vi "Dashboard Main.vi"() -> ()   [LabVIEW 2015]
uses:
  <vilib>/Utility/miscctls.llb/LVRowAndColumnTypeDef.ctl
  <vilib>/event_ctls.llb/eventvkey.ctl
  <vilib>/Rock Robotics/WPI/Dashboard/WPI_DashboardLogging Global.vi
  <vilib>/Rock Robotics/Network Tables/NT Read Numeric Array.vi
  <vilib>/Utility/config.llb/Write Key (String).vi
  <vilib>/Utility/config.llb/Write Key (I32).vi
  <vilib>/Utility/config.llb/NI_LVConfig.lvlib
panel:
  in  "TCP":refnum<k5>
  in  "Rec Mode":enum32{"Stop", "Record", "Playback"}(radio)
  in  "Vision":u16(ring) items=["Camera Off", "USB Camera SW", "USB Camera HW", "IP Camera"]
  out "Camera IP":string
  out "Image Message":string="Timeout in Camera Communications"
  in  "Dashboard Tab":T1(tab)
  out "dist":dbl
  in  "Select Auto":string(combo)
  out "NT Connection":bool
  in  "Camera Settings":T2={"Frame Rate"=30, "Compression"=30, "Size"=1} {"Frame Rate" scale=1.0..30.0; "Size" items=["640x480", "320x240", "160x120"]}
  out "MotorChart R":cluster{"Numeric":dbl, "Numeric":dbl}(graph)
  out "MotorChart L":T3(graph)
  out "MotorSliders R":cluster{"MotorSlide1":dbl, "MotorSlide2":dbl} {"MotorSlide2" scale=-1.0..1.0 scale format="%#_2e"; "MotorSlide1" scale=-1.0..1.0 scale format="%#_2e"}
  out "MotorSliders L":T4 {"MotorSlide4 2" scale=0.0..14.0 scale format="%#_2e"; "MotorSlide2" scale=-1.0..1.0 scale format="%#_2e"; "MotorSlide1" scale=-1.0..1.0 scale format="%#_2e"}
  out "Gyro":dbl(knob) scale=0.0..360.0
  out "JS1 Z":dbl(slide) scale=-1.0..1.0 scale format="%#_2e"
  out "JS1 Graph":cluster{"X":dbl, "Y":dbl}[](graph)
  out "JS1 Buttons":T5
  out "JS2 Z":dbl(slide) scale=-1.0..1.0 scale format="%#_2e"
  out "JS2 Graph":cluster{"X":dbl, "Y":dbl}[](graph)
  out "JS2 Buttons":T5
  out "Mode":T6(ring)=enum."Auto Disabled"
  in  "DB Camera Config":bool
  out "fps":dbl format="%#.1g"
  out "Mbps":dbl format="%#.1g"
  out "Mbps LED":bool
  in  "DB/String 9":string
  in  "DB/String 8":string
  in  "DB/String 7":string
  in  "DB/String 6":string
  in  "DB/String 5":string
  in  "DB/String 4":string
  in  "DB/String 3":string
  in  "DB/String 2":string
  in  "DB/String 1":string
  in  "DB/String 0":string
  in  "DB/Slider 0":dbl(slide) scale=0.0..5.0
  in  "DB/Slider 1":dbl(slide) scale=0.0..5.0
  in  "DB/Slider 2":dbl(slide) scale=0.0..5.0
  in  "DB/Slider 3":dbl(slide) scale=0.0..5.0
  out "DB/LED 3":bool
  out "DB/LED 2":bool
  out "DB/LED 1":bool
  out "DB/LED 0":bool
  in  "DB/Button 3":bool
  in  "DB/Button 2":bool
  in  "DB/Button 1":bool
  in  "DB/Button 0":bool caption="New Name"
  in  "Test Slider":dbl(slide) scale=0.0..100.0 scale format="%#_3g"
  in  "On/Off":bool caption="Solenoid"
  in  "Test Name":u16(ring) items=["Select the test to run..."]
  in  "Test Tree":string(tree)
  in  "Motor":cluster{"Value":dbl, "Enable":bool} {"Value" scale=-1.0..1.0 scale format="%#_3g"}
  out "Progress":T7 {"Test Progress" scale=0.0..100.0}
  in  "Rev/Fwd":cluster{"Forward":bool, "Reverse":bool}
  in  "Test Ring":u16(ring) items=["Monochrome", "Color"]
  out "Cmd Status":string
  in  "Execute Command":bool
  in  "Command Params":string[][](table)
  in  "Command Selection":i32(listbox)
  in  "CheckList":i32(listbox)
  out "Tree":string(tree)
  out "Camera Image":T8(plugin-control)
  out "Background":bool
  # "Left"
  # "Front"
  # "Right"
  # "Battery"
  # "This tab is a great place for autonomous settings and robot-specific values.\nPlace controls and indicators inside this tab and match name to\nDashboard Variables on robot. You can also delete this comment."
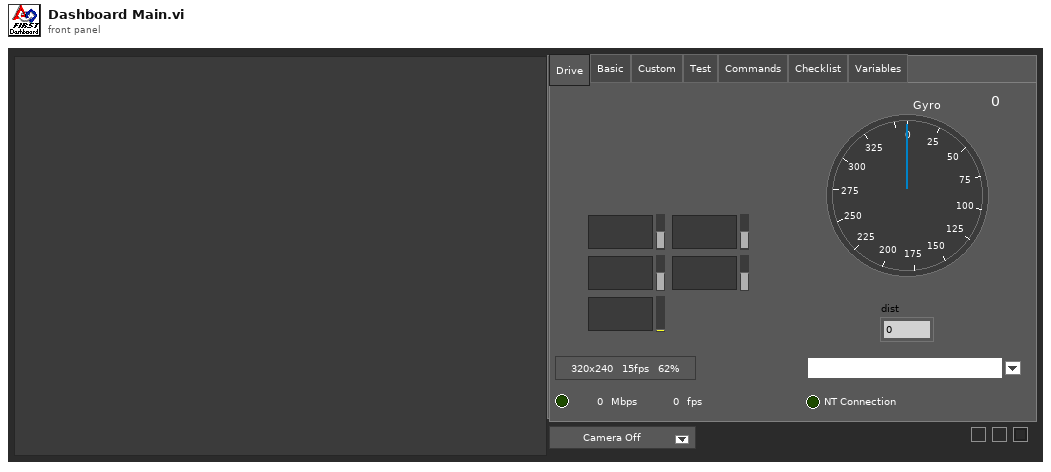
[diagram p1: front panel]
types:
  T1 = enum32{"Drive", "Basic", "Custom", "Test", "Commands", "Checklist", "Variables"}
  T2 = cluster{"Frame Rate":i32, "Compression":i32, "Size":u16}
  T3 = cluster{"Numeric":dbl, "Numeric":dbl, "Battery V":dbl}
  T4 = cluster{"MotorSlide1":dbl, "MotorSlide2":dbl, "MotorSlide4 2":dbl}
  T5 = cluster{bool, bool, bool, bool, bool, bool, bool, bool, bool, bool, bool, bool}
  T6 = enum8{"Tele-Op Disabled", "Tele-Op Enabled", "Auto Disabled", "Auto Enabled", "Test Disabled", "Test Enabled", "Disconnected", "No Code", "E-Stop"}
  T7 = cluster{"Test Progress":u8, "Test Progress Text":string}
  T8 = typedef "IMAQ Image.ctl" = refnum<image>
  T9 = cluster{"IDs":cluster{"RPC field ID":u16, "Unique ID":u16}, "String":string}
  T10 = enum32{"Drive", "Basic", "Custom", "Test", "Checklist", "Variables"}
  T11 = typedef "Image Type" = u32
  T12 = cluster{"Camera Image":refnum<vi>, "Dashboard Tab":refnum<vi>, "Background":refnum<vi>, "Vision":refnum<vi>, "Rec Mode":refnum<vi>, "Test Slider":refnum<vi>, "On/Off ":refnum<vi>, "Test Ring":refnum<vi>, "Rev/Fwd":refnum<vi>, "Test Name":refnum<vi>, "Motor":refnum<vi>, "Progress":refnum<vi>, "CheckList":refnum<vi>, "Tree":refnum<vi>, "Test Tree":refnum<vi>, "Command Params":refnum<vi>, "Command Selection":refnum<vi>, "Execute Command":refnum<vi>, "Cmd Status":refnum<vi>}
  T13 = cluster{"Error Strings":string, "Disable Counts":cluster{u16, u16}, "Rail Faults":cluster{u16, u16, u16}, "Robot IP":string, "DB Mode":u8, "Event Info":cluster{"Name":string, "Type":u8, "Number":u16, "Replay":u8}, "Camera Addr":string}
  T14 = cluster{"Storage":cluster{"Disk Free":u64, "RAM Block":u32, "RAM free":u32}, "CPU Utilization":cluster{"CPU % ISR":sgl, "CPU % Time Crit":sgl, "CPU % Timed Str":sgl, "CPU % High":sgl, "CPU % Above":sgl, "CPU % Normal":sgl, "CPU % Low":sgl}, "CAN":cluster{"% Bus Utilization":sgl, "Bus Off Cnt":u32, "TX_FIFO Full Cnt":u32, "Receive Error Cnt":u8, "Transmit Error Cnt":u8}, "HID":cluster{"HID Outputs":u32, "Rumble Low":u16, "Rumble High":u16}[]}
  T15 = cluster{"Status bits":cluster{"Test Mode":bool, "Autonomous":bool, "Enabled":bool, "Code Start":bool, "Brownout":bool, "Reserved 2":bool, "Reserved 3":bool, "E-Stop":bool}, "Code Trace":cluster{"Disabled":bool, "TeleOp":bool, "Auto":bool, "Test":bool}, "Controller Type":enum16{"unknown", "cRIO", "roboRio"}, "Code?":enum16{"unknown", "noCode", "code"}, "Battery V":dbl}
  T16 = cluster{"Control Bits":cluster{"TestMode":bool, "Autonomous":bool, "Enabled":bool, "FMS Present":bool, bool, bool, bool, "E-Stop":bool}, "Team Station ":u8, "Countdown":sgl, "Joystick Values":cluster{"Axes":dbl[], "Buttons":bool[], "POVs":i16[]}[]}
  T17 = cluster{"Axes":dbl[], "Buttons":bool[], "POVs":i16[]}[]
  T18 = cluster{"Axes":dbl[], "Buttons":bool[], "POVs":i16[]}
  T19 = cluster{"Buttons[0]":bool, "Buttons[1]":bool, "Buttons[2]":bool, "Buttons[3]":bool, "Buttons[4]":bool, "Buttons[5]":bool, "Buttons[6]":bool, "Buttons[7]":bool, "Buttons[8]":bool, "Buttons[9]":bool, "Buttons[10]":bool, "Buttons[11]":bool}
  T20 = typedef "NI_LVConfig.lvlib/Config Data RefNum.ctl" = refnum<k1>
  T21 = cluster{"Operation":enum16{"Update", "Clear"}, "Color Box":u32}[]
  T22 = typedef "eventvkey.ctl" = enum16{"ASCII", "Enter", "Return", "Shift", "Ctrl", "Alt", "Cmd", "Opt", "Caps", "NumLock", "Clear", "Break", "Up", "Down", "Left", "Right", "Insert", "Delete", "Home", "End", "PageUp", "PageDown", "Escape", "Help", "Pause", "ScrollLock", "F1", "F2", "F3", "F4", "F5", "F6", "F7", "F8", "F9", "F10", "F11", "F12", "F13", "F14", "F15", "F16", "F17", "F18", "F19", "F20", "F21", "F22", "F23", "F24", "Play", "VolumeUp", "VolumeDown", "Mute", "Two Byte Char"}
  T23 = cluster{"Image Size":bool, "Image Type":bool, "Pixel Value":bool, "ROI Information":bool, "Zoom Factor":bool}
  T24 = enum8{"Enabled", "Disabled", "Disabled and Grayed Out"}
  T25 = cluster{"Operation":enum16{"Update", "Clear"}, "Color Box":u32}
  T26 = typedef "LVRowAndColumnTypeDef.ctl" = cluster{"Row":i32, "Column":i32}
  T27 = cluster{"Shift":bool, "Ctrl":bool, "Alt":bool, "Cmd":bool, "Opt":bool}
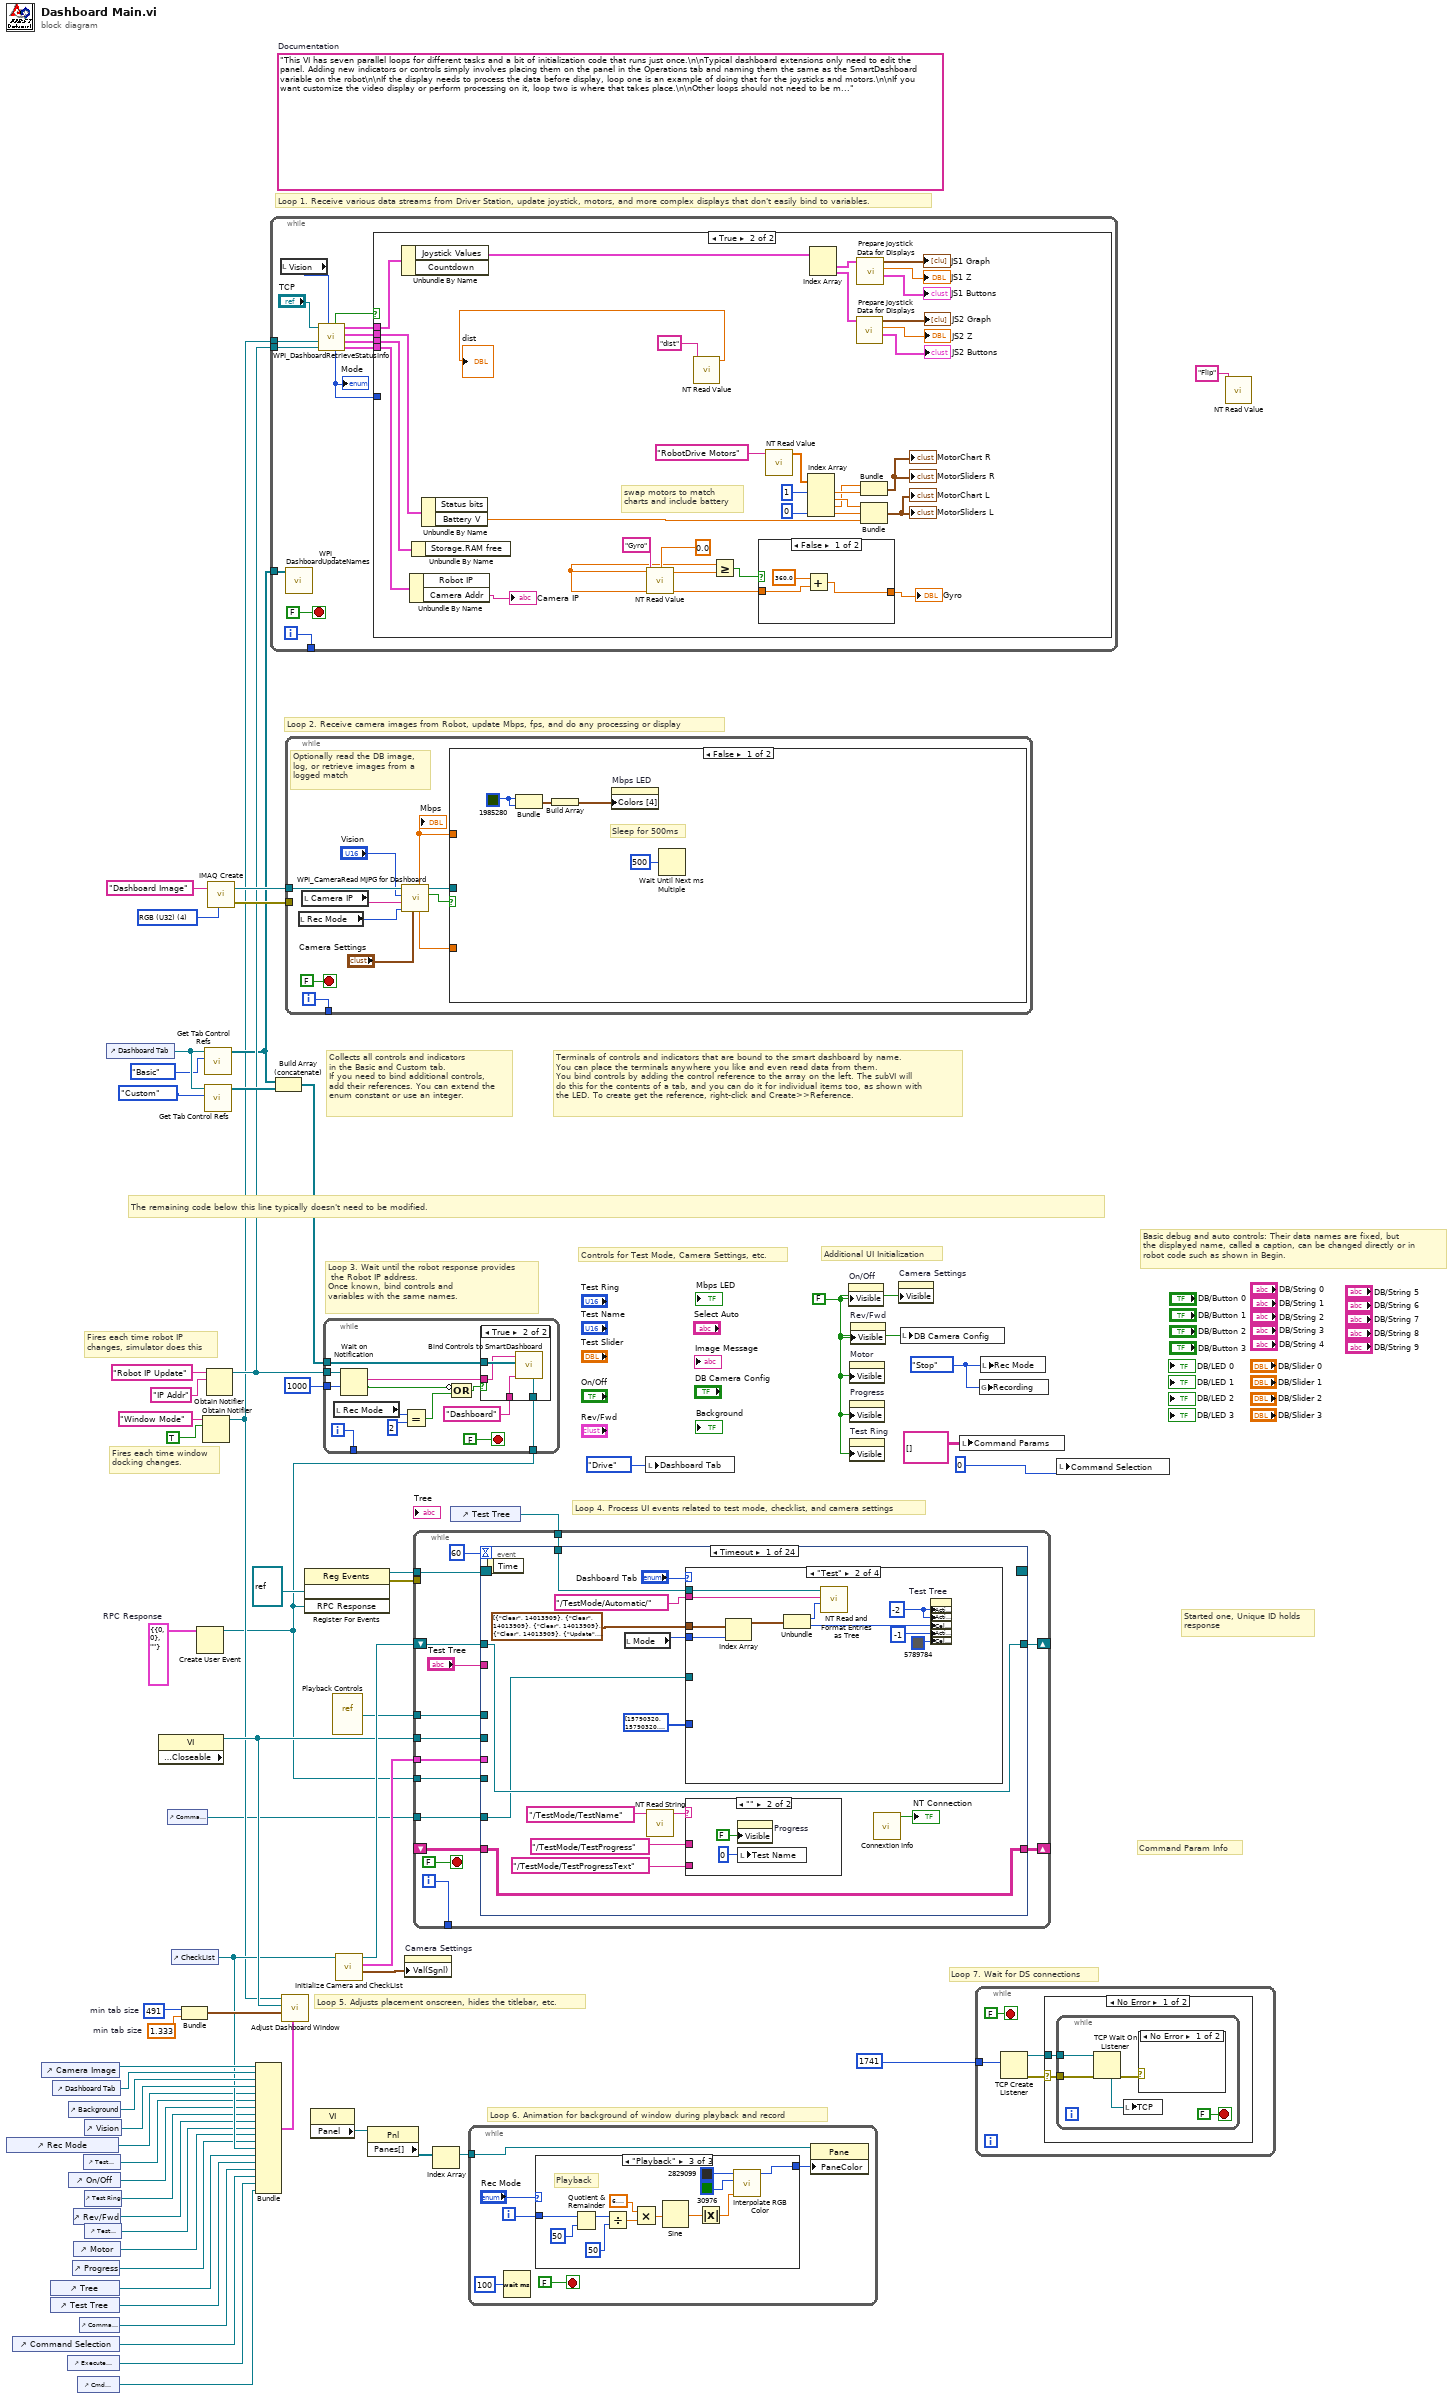
[diagram p0: block diagram]
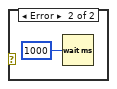
[diagram p2: hidden frame]
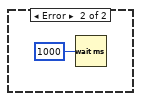
[diagram p3: hidden frame]
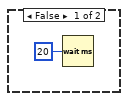
[diagram p4: hidden frame]
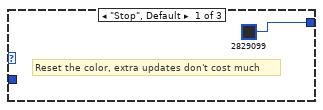
[diagram p6: hidden frame]
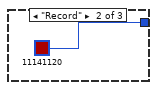
[diagram p7: hidden frame]
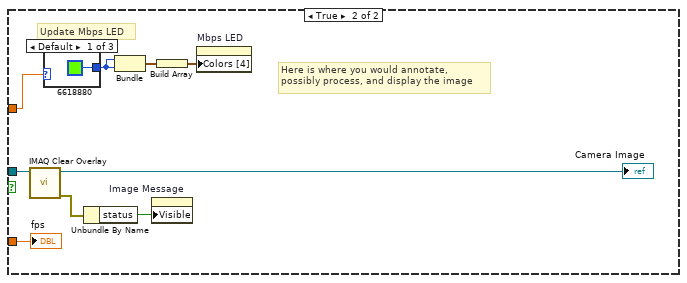
[diagram p9: hidden frame]
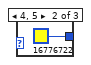
[diagram p10: hidden frame]
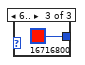
[diagram p11: hidden frame]
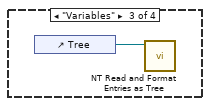
[diagram p13: hidden frame]
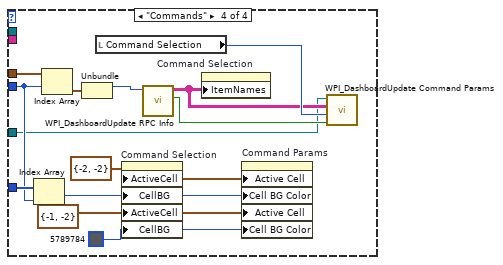
[diagram p14: hidden frame]
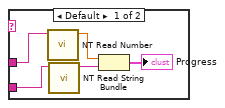
[diagram p15: hidden frame]
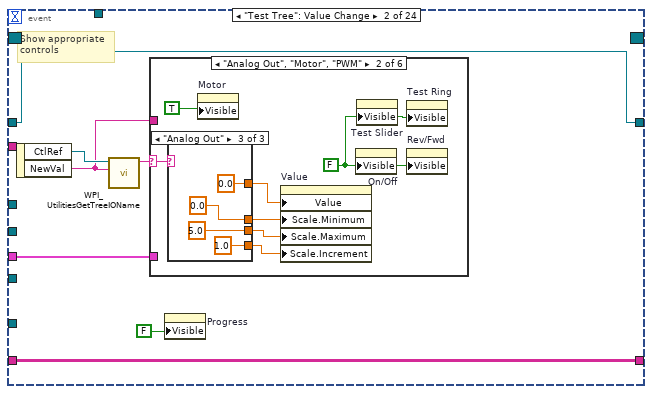
[diagram p16: hidden frame]
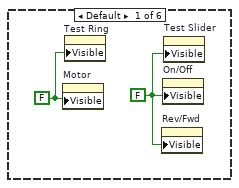
[diagram p17: hidden frame]
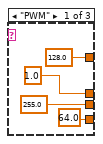
[diagram p18: hidden frame]
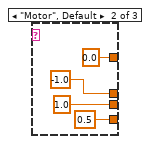
[diagram p19: hidden frame]
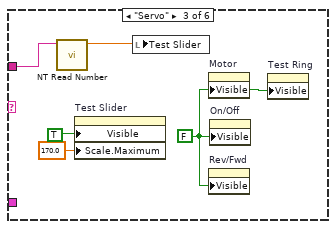
[diagram p20: hidden frame]
diagram:
  w8 = T9 {"IDs"={"RPC field ID"=0, "Unique ID"=0}, "String"=""}  # RPC Response
  w34 = 491  # min tab size
  w33 = 1.333  # min tab size
  w42 = enum32{"Stop", "Record", "Playback"}."Stop" ("Rec Mode")
  w16 = FALSE ("Visible")
  (unwired) "This VI has seven parallel loops for different tasks and a bit of initialization code that runs just once.\n\nTypical dashboard extensions only need to edit the panel. Adding new indicators or controls simply involves placing them on the panel in the Operations tab and naming them the same as the SmartDashboard variable on the robot\n\nIf the display needs to process the data before display, loop one is an example of doing that for the joysticks and motors.\n\nIf you want customize the video display or perform processing on it, loop two is where that takes place.\n\nOther loops should not need to be modified. They are pretty standard, and document the task they perform."  # Documentation
  w62 = T11 4 items=["Grayscale (U8)", "Grayscale (I16)", "Grayscale (SGL)", "Complex (CSG)", "RGB (U32)", "HSL (U32)", "RGB (U64)"] ("Image Type")
  # "Command Param Info"
  # "Started one, Unique ID holds\nresponse"
  # "Loop 7. Wait for DS connections"
  # "Basic debug and auto controls: Their data names are fixed, but\nthe displayed name, called a caption, can be changed directly or in\nrobot code such as shown in Begin."
  # "Controls for Test Mode, Camera Settings, etc."
  # "Additional UI Initialization"
  # "Loop 6. Animation for background of window during playback and record"
  # "Fires each time robot IP\nchanges, simulator does this"
  # "Fires each time window\ndocking changes."
  # "Collects all controls and indicators\nin the Basic and Custom tab.\nIf you need to bind additional controls,\nadd their references. You can extend the\nenum constant or use an integer."
  # "The remaining code below this line typically doesn't need to be modified."
  # "Loop 4. Process UI events related to test mode, checklist, and camera settings"
  # "Terminals of controls and indicators that are bound to the smart dashboard by name.\nYou can place the terminals anywhere you like and even read data from them.\nYou bind controls by adding the control reference to the array on the left. The subVI will\ndo this for the contents of a tab, and you can do it for individual items too, as shown with\nthe LED. To create get the reference, right-click and Create>>Reference."
  # "Loop 3. Wait until the robot response provides\n the Robot IP address.\nOnce known, bind controls and\nvariables with the same names."
  # "Loop 5. Adjusts placement onscreen, hides the titlebar, etc."
  # "Loop 1. Receive various data streams from Driver Station, update joystick, motors, and more complex displays that don't easily bind to variables."
  # "Loop 2. Receive camera images from Robot, update Mbps, fps, and do any processing or display"
  n1 = control-ref of="Rec Mode"() -> (w22:refnum<vi>)
  n2 = control-ref of="Command Selection"() -> (w7:refnum<vi>)
  n3 = control-ref of="Camera Image"() -> (w37:refnum<vi>)
  n4 = control-ref of="Tree"() -> (w26:refnum<vi>)
  n5 = control-ref of="Test Tree"() -> (w25:refnum<vi>)
  n6 = control-ref of="Dashboard Tab"() -> (w36:refnum<vi>)
  n7 = control-ref of="Execute Command"() -> (w9:refnum<vi>)
  n8 = control-ref of="Background"() -> (w31:refnum<vi>)
  n9 = control-ref of="On/Off"() -> (w20:refnum<vi>)
  n10 = control-ref of="Progress"() -> (w17:refnum<vi>)
  n11 = control-ref of="Rev/Fwd"() -> (w18:refnum<vi>)
  n12 = control-ref of="Motor"() -> (w23:refnum<vi>)
  n13 = control-ref of="Cmd Status"() -> (w3:refnum<vi>)
  n14 = control-ref of="Command Params"() -> (w10:refnum<vi>)
  n15 = control-ref of="Test Slider"() -> (w21:refnum<vi>)
  n16 = control-ref of="Vision"() -> (w35:refnum<vi>)
  n17 = control-ref of="Test Ring"() -> (w19:refnum<vi>)
  n18 = control-ref of="Test Name"() -> (w24:refnum<vi>)
  n19 = control-ref of="Dashboard Tab"() -> (w40:refnum<vi>)
  n20 = property class="VI" props=["Front Panel.Closeable"]() -> (reference out=w41:refnum<vi>)  [unwired: 2 in, 2 out]
  n21 = control-ref of="Command Params"() -> (w2:refnum<vi>)
  n22 = control-ref of="CheckList"() -> (w27:refnum<vi>)
  n23 = Bundle("min tab size"=w34, "min tab size"=w33) -> (w32:cluster{"min tab size":i32, "min tab size":dbl})  [unwired: 1 in]
  n24 = Create User Event(user event datatype=w8) -> (user event=w4:refnum<user-event>)  [unwired: 1 in, 1 out]
  n25 = Obtain Notifier(name (unnamed)="Window Mode", notification data type=TRUE) -> (notifier out=w13:refnum<notifier>)  [unwired: 2 in, 2 out]
  n26 = call <vilib>:"Get Tab Control Refs.vi"("Page Index"=T10."Basic" ("Dashboard Tab"), "TabControl in"=w40) -> ("ControlsOnPage"=w14:refnum<vi>[])  [unwired: 9 in]
  n27 = call <vilib>:"Get Tab Control Refs.vi"("Page Index"=T10."Custom" ("Dashboard Tab"), "TabControl in"=w40) -> ("ControlsOnPage"=w39:refnum<vi>[])  [unwired: 9 in]
  n28 = Obtain Notifier(name (unnamed)="Robot IP Update", notification data type="IP Addr" ("name (unnamed)")) -> (notifier out=w15:refnum<notifier>)  [unwired: 2 in, 2 out]
  n29 = call "IMAQ Create"("Image Name"="Dashboard Image", "Image Type"=w62) -> ("New Image"=w60:T8, "error out"=w59:errorcluster)  [unwired: 2 in, 1 out]
  n30 = Bundle("Camera Image"=w37, "Dashboard Tab"=w36, "Background"=w31, "Vision"=w35, "Rec Mode"=w22, "Test Slider"=w21, "On/Off"=w20, "Test Ring"=w19, "Rev/Fwd"=w18, "Test Name"=w24, "Motor"=w23, "Progress"=w17, "CheckList"=w27, "Tree"=w26, "Test Tree"=w25, "Command Params"=w10, "Command Selection"=w7, "Execute Command"=w9, "Cmd Status"=w3) -> (w28:T12)  [unwired: 1 in]
  n31 = while {
    tunnel: [w74] -> _
    tunnel: w15 -> [w68]
    tunnel: w14 -> [w67]
    tunnel: w13 -> [w63]
    i -> [w74]
    stop <- FALSE stop-if-true
    n32 = local read "Vision"() -> (w65:u16)
    n33 = call <vilib>:"WPI_DashboardUpdateNames.vi"("Controls on Tab"=w67) -> ()  [unwired: 11 in]
    n34 = call <vilib>:"WPI_DashboardRetrieveStatusInfo.vi"("Vision"=w65, "Binding Refnum"=w68, "Window Mode Notifier"=w63, "TCP Cnx"="TCP") -> ("Power and Errors"=w69:T13, "Robot Metrics"=w72:T14, "Status Info"=w73:T15, "Control Info"=w70:T16, "Robot Mode"=w66:T6, "Process?"=w71:bool)  [unwired: 2 in]
    "Mode" <- w66
    n35 = case shown="True" w71 {
      tunnel: w73 -> [_ w108]
      tunnel: w72 -> [_ w107]
      tunnel: w70 -> [_ w106]
      tunnel: w69 -> [_ w105]
      tunnel: w66 -> [_ _]
      frame False {
        n36 = Wait (ms)(milliseconds to wait=u32 20) -> ()  [unwired: 1 out]
      }
      frame True {
        # "swap motors to match\ncharts and include battery"
        n37 = Unbundle By Name(w106) -> ("Joystick Values"=w95:T17)  [unwired: 1 out]
        n38 = Unbundle By Name(w105) -> ("Camera Addr"=→"Camera IP":string)  [unwired: 1 out]
        n39 = Unbundle By Name(w107) -> ()  [unwired: 1 out]
        n40 = Unbundle By Name(w108) -> ("Battery V"=w96:dbl)  [unwired: 1 out]
        n41 = call-poly <vilib>:"NT Read Value.vi"("Name"="Gyro") -> ("Numeric"=w80:dbl)  [unwired: 9 in, 1 out]
        n42 = call-poly <vilib>:"NT Read Value.vi"("Name"="dist") -> ("Numeric"=→"dist":dbl)  [unwired: 9 in, 1 out]
        n43 = Greater Or Equal?(x=w80, y=0.0) -> (x >= y?=w82:bool)
        n44 = case shown="False" w82 {
          tunnel: [w109 w112] -> w79
          tunnel: w80 -> [w110 w112]
          frame False {
            n45 = Add(x=360.0, y=w110) -> (x+y=w109:dbl)
          }
          frame True {
          }
        }
        "Gyro" <- w79
        n46 = call-poly <vilib>:"NT Read Value.vi"("Name"="RobotDrive Motors") -> ("Numeric Array"=w84:dbl[])  [unwired: 9 in, 1 out]
        n47 = Index Array(array=w84, index #1=1, index #4=0) -> (element #1=w100:dbl, element #2=w101:dbl, element #3=w99:dbl, element #4=w104:dbl)  [unwired: 2 in]
        n48 = Index Array(array=w95) -> (element #1=w94:T18, element #2=w89:T18)  [unwired: 2 in]
        n49 = call "Prepare Joystick Data for Displays.vi"("Joystick Values"=w89) -> ("Buttons"=→"JS2 Buttons":T19, "Z Axis"=→"JS2 Z":dbl, "Cartesian Data"=→"JS2 Graph":cluster{"X axis":dbl, "X axis":dbl}[])  [unwired: 8 in]
        n50 = call "Prepare Joystick Data for Displays.vi"("Joystick Values"=w94) -> ("Buttons"=→"JS1 Buttons":T19, "Z Axis"=→"JS1 Z":dbl, "Cartesian Data"=→"JS1 Graph":cluster{"X axis":dbl, "X axis":dbl}[])  [unwired: 8 in]
        n51 = Bundle("Numeric"=w99, "Numeric"=w100) -> (→"MotorChart R" →"MotorSliders R":cluster{"Numeric":dbl, "Numeric":dbl})  [unwired: 1 in]
        n52 = Bundle("Numeric"=w101, "Numeric"=w104, "Battery V"=w96) -> (→"MotorChart L" →"MotorSliders L":T3)  [unwired: 1 in]
      }
    }
  }
  n53 = Build Array (concatenate)(w14, w39) -> (w38:refnum<vi>[])
  n54 = call "Adjust Dashboard Window.vi"("Sizing Refnums"=w28, "Size Constraints"=w32, "VI"=w41, "WIn Mode"=w13) -> ()  [unwired: 8 in]
  n55 = while {
    tunnel: w60 -> [w121]
    tunnel: w59 -> [_]
    tunnel: [w122] -> _
    i -> [w122]
    stop <- FALSE stop-if-true
    # "Optionally read the DB image,\nlog, or retrieve images from a\nlogged match"
    n56 = local read "Rec Mode"() -> (w116:enum32{"Stop", "Record", "Playback"})
    n57 = local read "Camera IP"() -> (w114:string)
    n58 = call <vilib>:"WPI_CameraRead MJPG for Dashboard.vi"("Camera Settings"="Camera Settings", "Rec Mode"=w116, "Camera IP"=w114, "Camera Mode"="Vision", "Refnum in"=w121) -> ("Active"=w119:bool, "Refnum out"=w120:T8, "FPS"=w118:dbl, "Bandwidth (Mbps)"=w113:dbl)  [unwired: 3 in]
    "Mbps" <- w113
    n59 = case shown="False" w119 {
      tunnel: w120 -> [_ w131]
      tunnel: w113 -> [_ w130]
      tunnel: w118 -> [_ w128]
      frame False {
        w124 = u32 1985280 ("Color Box")
        # "Sleep for 500ms"
        n60 = Bundle("Color Box"=w124, "Color Box"=w124) -> (w126:cluster{"Color Box":u32, "Color Box":u32})  [unwired: 1 out]
        n61 = Build Array(w126) -> (w125:cluster{"Color Box":u32, "Color Box":u32}[])
        n62 = property on="Mbps LED" class="Bool (strict)"("Colors [4]"=w125) -> ()  [unwired: 2 in, 2 out]
        n63 = Wait Until Next ms Multiple(millisecond multiple=u32 500) -> ()  [unwired: 1 out]
      }
      frame True {
        # "Here is where you would annotate,\npossibly process, and display the image"
        # "Update Mbps LED"
        n64 = call "IMAQ Clear Overlay"("Image"=w131) -> ("error out"=w135:errorcluster, "Image Out"=→"Camera Image":T8)  [unwired: 2 in, 7 out]
        n65 = case shown="Default" w130 {
          tunnel: [u32 6618880 ("Color Box") u32 16776722 ("Color Box") u32 16716800 ("Color Box")] -> w132
          frame Default {
          }
          frame 4, 5 {
          }
          frame 6.. {
          }
        }
        n66 = Unbundle By Name(w135) -> ("status"=w136:bool)
        n67 = Bundle("Color Box"=w132, "Color Box"=w132) -> (w134:cluster{"Color Box":u32, "Color Box":u32})  [unwired: 1 out]
        n68 = property on="Image Message" class="Str"("Visible"=w136) -> ()  [unwired: 2 in, 2 out]
        n69 = Build Array(w134) -> (w133:cluster{"Color Box":u32, "Color Box":u32}[])
        n70 = property on="Mbps LED" class="Bool (strict)"("Colors [4]"=w133) -> ()  [unwired: 2 in, 2 out]
        "fps" <- w128
      }
    }
  }
  n71 = register-events(refnum<vi> refnum, w4) -> (reference out=w46:refnum<event-registration>, error out=w45:errorcluster)  [unwired: 2 in]
  n72 = property class="VI"() -> ("Panel"=w49:refnum<vi>)  [unwired: 2 in, 2 out]
  n73 = while {
    tunnel: w38 -> [w152]
    tunnel: w15 -> [w150]
    tunnel: [w148] -> _
    tunnel: u32 1000 ("milliseconds to wait") -> [w147]
    tunnel: w4 -> [w140]
    i -> [w148]
    stop <- FALSE stop-if-true
    n74 = local read "Rec Mode"() -> (w143:enum32{"Stop", "Record", "Playback"})
    n75 = Wait on Notification(notifier=w150, timeout in ms (-1)=w147) -> (notification=w149:string, timed out?=w145:bool)  [unwired: 2 in, 2 out]
    n76 = Equal?(x=w143, y=u16 2 ("Rec Mode")) -> (x = y?=w144:bool)
    n77 = Compound Arithmetic op=OR(invert w145, w144) -> (w146:bool)
    n78 = case shown="True" w146 {
      tunnel: w152 -> [_ w156]
      tunnel: w149 -> [_ w155]
      tunnel: "Dashboard" -> [_ w154]
      tunnel: w140 -> [_ w153]
      frame False {
      }
      frame True {
        n79 = call <vilib>:"Bind Controls to SmartDashboard.vi"("RPC ref"=w153, "Client Name"=w154, "Bound Control Refs"=w156, "Server IP Address"=w155) -> ()  [unwired: 8 in]
      }
    }
  }
  n80 = vi-ref "Playback Controls.vi"() -> (w47:refnum<vi>)
  n81 = call "Initialize Camera and CheckList.vi"("ListBox in"=w27) -> ("Cluster"=w53:cluster{"value":i32, "value":i32, "index":i32}, "Array"=w54:cluster{string[]}[], "File Refnum"=w52:T20)  [unwired: 8 in]
  n82 = property class="Pnl"(reference=w49) -> ("Panes[]"=w50:refnum<vi>[])  [unwired: 1 in, 2 out]
  n83 = property on="Camera Settings" class="Clust (strict)"("Val(Sgnl)"=w53) -> ()  [unwired: 2 in, 2 out]
  n84 = Index Array(array=w50) -> (element=w48:refnum<vi>)  [unwired: 1 in]
  n85 = control-ref of="Test Tree"() -> (w51:refnum<vi>)
  n86 = while {
    tunnel: w54 -> [w168]
    shift-right: [w167] -> _
    shift-left: w52 -> [w166]
    tunnel: [w165] -> _
    tunnel: w51 -> [w164]
    tunnel: w47 -> [w163]
    tunnel: w46 -> [w162]
    tunnel: w45 -> [_]
    tunnel: w41 -> [w161]
    tunnel: w4 -> [w160]
    tunnel: w2 -> [w159]
    shift-right: [w158] -> _
    shift-left: _ -> [w157]
    i -> [w165]
    stop <- FALSE stop-if-true
    n87 = event shown="[0] Timeout" {
      selector: w162 -> [_ _ _ _ _ _ _ _ _ _ _ _ _ _ _ _ _ _ _ _ _ _ _ _]
      dyn-events: [_ _ _ _ _ _ _ _ _ _ _ _ _ _ _ _ _ _ w477 _ _ _ _ _] -> _
      timeout: u32 60 ("milliseconds to wait") -> [_ _ _ _ _ _ _ _ _ _ _ _ _ _ _ _ _ _ _ _ _ _ _ _]
      tunnel: w164 -> [w181 _ _ _ _ _ _ _ _ _ _ _ _ _ _ _ _ _ _ _ _ _ _ _]
      tunnel: "Test Tree" -> [_ _ _ _ _ _ _ _ _ _ _ _ _ w440 w449 w452 w457 w466 _ _ _ _ _ _]
      tunnel: w168 -> [_ w219 _ _ _ _ _ _ _ _ _ w402 w433 _ _ _ _ _ _ _ _ _ _ _]
      tunnel: [w178 w218 w322 w328 w338 w342 w348 w360 w368 w374 w387 w401 w426 w439 w447 w451 w456 w465 w479 w495 w497 w505 w516 w521] -> w167
      tunnel: w166 -> [w178 w218 w322 w328 w338 w342 w348 w360 w368 w374 w387 w400 w426 w439 w447 w451 w456 w465 w479 w495 w497 w505 w516 w521]
      tunnel: w163 -> [_ _ _ _ _ _ _ _ _ _ _ _ _ _ _ _ _ _ w480 _ w500 _ _ _]
      tunnel: w161 -> [_ _ _ _ _ _ _ _ _ _ _ _ _ _ _ _ _ _ w475 _ _ _ _ _]
      tunnel: w160 -> [_ _ _ _ _ _ _ _ _ _ _ _ _ _ _ _ _ _ w471 _ _ _ _ _]
      tunnel: w159 -> [w173 _ _ _ _ _ w346 _ _ _ _ _ _ _ _ _ _ _ _ _ _ _ _ _]
      tunnel: [w172 w217 w321 w327 w337 w343 w344 w354 w365 w373 w386 w399 w425 w438 w446 w450 w455 w464 w470 w493 w496 w501 w509 w522] -> w158
      tunnel: w157 -> [w172 w217 w321 w327 w337 w343 w344 _ _ w373 w386 w399 w425 w438 w446 w450 w455 w464 w470 w493 w496 w501 w509 w522]
      event Timeout {
        n88 = event-data() -> ()  [unwired: 1 in, 1 out]
        n89 = local read "Mode"() -> (w175:T6)
        n90 = call <vilib>:"NT Read String.vi"("Name"="/TestMode/TestName") -> ("String"=w184:string)  [unwired: 9 in, 1 out]
        n91 = case shown="\"Test\"" "Dashboard Tab" {
          tunnel: w181 -> [_ w195 _ _]
          tunnel: "/TestMode/Automatic/" ("Name Pattern") -> [_ w194 _ _]
          tunnel: T21 [{"Operation"=enum."Clear", "Color Box"=14013909}, {"Operation"=enum."Clear", "Color Box"=14013909}, {"Operation"=enum."Clear", "Color Box"=14013909}, {"Operation"=enum."Clear", "Color Box"=14013909}, {"Operation"=enum."Update", "Color Box"=14013909}, {"Operation"=enum."Update", "Color Box"=16777215}, {"Operation"=enum."Clear", "Color Box"=14013909}, {"Operation"=enum."Clear", "Color Box"=14013909}, {"Operation"=enum."Clear", "Color Box"=14013909}] -> [_ w187 _ w204]
          tunnel: w175 -> [_ w186 _ w203]
          tunnel: u32[] [15790320, 15790320, 15790320, 15790320, 16777215, 16777215, 15790320, 15790320, 15790320] -> [_ _ _ w209]
          tunnel: w173 -> [_ _ _ w197]
          frame "Custom", Default {
          }
          frame "Test" {
            w193 = -2 ("Active Item:Row Number")
            n92 = Index Array(array=w187, index=w186) -> (element=w188:T25)
            n93 = Unbundle(w188) -> ("Operation"=w189:enum16{"Update", "Clear"}, "Color Box"=w190:u32)
            n94 = call <vilib>:"NT Read and Format Entries as Tree.vi"("Operation"=w189, "Name Pattern"=w194, "Tree Refnum"=w195) -> ()  [unwired: 7 in, 2 out]
            n95 = property on="Test Tree" class="Tree (strict)"("Active Item Row Number"=w193, "ActiveColNum"=w193, "CellBG"=w190, "Active Item Row Number"=-1 ("Active Item:Row Number"), "CellBG"=u32 5789784 ("Color Box")) -> ()  [unwired: 2 in, 2 out]
          }
          frame "Variables" {
            n96 = control-ref of="Tree"() -> (w196:refnum<vi>)
            n97 = call <vilib>:"NT Read and Format Entries as Tree.vi"("Tree Refnum"=w196) -> ()  [unwired: 9 in, 2 out]
          }
          frame "Commands" {
            w205 = u32 5789784 ("Color Box")
            w206 = T26 {"Row"=-1, "Column"=-2} ("Active Cell:Active Cell")
            w208 = T26 {"Row"=-2, "Column"=-2} ("Active Cell:Active Cell")
            n98 = Index Array(array=w209, index=w203) -> (element=w207:u32)
            n99 = Index Array(array=w204, index=w203) -> (element=w202:T25)
            n100 = Unbundle(w202) -> ("Operation"=w201:enum16{"Update", "Clear"})  [unwired: 1 out]
            n101 = local read "Command Selection"() -> (w200:i32)
            n102 = property on="Command Selection" class="MCListbox (strict)"("ActiveCell"=w208, "CellBG"=w207, "ActiveCell"=w206, "CellBG"=w205) -> ()  [unwired: 2 in, 2 out]
            n103 = call <vilib>:"WPI_DashboardUpdate RPC Info.vi"("Operation"=w201) -> ("update"=w199:bool, "commands"=w198:string[][])  [unwired: 9 in]
            n104 = property on="Command Selection" class="MCListbox (strict)"("ItemNames"=w198) -> ()  [unwired: 2 in, 2 out]
            n105 = property on="Command Params" class="Tbl (strict)"("Active Cell"=w208, "Cell BG Color"=w207, "Active Cell"=w206, "Cell BG Color"=w205) -> ()  [unwired: 2 in, 2 out]
            n106 = call <vilib>:"WPI_DashboardUpdate Command Params.vi"("Update"=w199, "NewVal"=w200, "Commands"=w198, "Param Tbl"=w197) -> ()  [unwired: 7 in, 1 out]
          }
        }
        n107 = case shown="\"\"" w184 {
          tunnel: "/TestMode/TestProgress" ("Name") -> [w211 _]
          tunnel: "/TestMode/TestProgressText" ("Name") -> [w210 _]
          frame Default {
            n108 = call <vilib>:"NT Read Number.vi"("Name"=w211) -> ("Numeric"=w212:dbl)  [unwired: 9 in, 1 out]
            n109 = call <vilib>:"NT Read String.vi"("Name"=w210) -> ("String"=w213:string)  [unwired: 9 in, 1 out]
            n110 = Bundle("Numeric"=w212, "String"=w213) -> (→"Progress":cluster{"Numeric":dbl, "String":string})  [unwired: 1 in]
          }
          frame "" {
            n111 = property on="Progress" class="Clust (strict)"("Visible"=FALSE) -> ()  [unwired: 2 in, 2 out]
            n112 = local write "Test Name"(u16 0) -> ()
          }
        }
        n113 = call <vilib>:"Connextion Info.vi"() -> ("Connected"=→"NT Connection":bool)  [unwired: 10 in, 1 out]
      }
      event "Test Tree": Value Change {
        # "Show appropriate\ncontrols"
        n114 = event-data() -> ("CtlRef"=w222:refnum<vi>, "NewVal"=w220:string)  [unwired: 1 in]
        n115 = call <vilib>:"WPI_UtilitiesGetTreeIOName.vi"("NewVal"=w220, "TreeControl in"=w222) -> ("I/O Name"=w223:string)  [unwired: 9 in]
        n116 = case shown="\"Analog Out\", \"Motor\", \"PWM\"" w223 {
          selector: w223 -> [_ w230 _ w252 w261 _]
          tunnel: w220 -> [_ _ w249 w251 _ w268]
          tunnel: w219 -> [_ _ _ _ _ w267]
          frame Default {
            w225 = FALSE ("Visible")
            w224 = FALSE ("Visible")
            n117 = property on="Motor" class="Clust (strict)"("Visible"=w224) -> ()  [unwired: 2 in, 2 out]
            n118 = property on="Test Ring" class="Ring (strict)"("Visible"=w224) -> ()  [unwired: 2 in, 2 out]
            n119 = property on="Rev/Fwd" class="Clust (strict)"("Visible"=w225) -> ()  [unwired: 2 in, 2 out]
            n120 = property on="On/Off" class="Bool (strict)"("Visible"=w225) -> ()  [unwired: 2 in, 2 out]
            n121 = property on="Test Slider" class="Slide (strict)"("Visible"=w225) -> ()  [unwired: 2 in, 2 out]
          }
          frame "Analog Out", "Motor", "PWM" {
            w231 = FALSE ("Visible")
            n122 = case shown="\"Analog Out\"" w230 {
              tunnel: [1.0 ("Value") -1.0 ("Value") 0.0 ("Value")] -> w229
              tunnel: [255.0 ("Value") 1.0 ("Value") 5.0 ("Value")] -> w228
              tunnel: [128.0 ("Value") 0.0 ("Value") 0.0 ("Value")] -> w227
              tunnel: [64.0 ("Value") 0.5 ("Value") 1.0 ("Value")] -> w226
              frame "PWM" {
              }
              frame "Motor", Default {
              }
              frame "Analog Out" {
              }
            }
            n123 = property on="Motor" class="Clust (strict)"("Visible"=TRUE) -> ()  [unwired: 2 in, 2 out]
            n124 = property on="Value" class="Slide (strict)"("Value"=w227, "Scale.Minimum"=w229, "Scale.Maximum"=w228, "Scale.Increment"=w226) -> ()  [unwired: 2 in, 2 out]
            n125 = property on="On/Off" class="Bool (strict)"("Visible"=w231) -> ()  [unwired: 2 in, 2 out]
            n126 = property on="Test Slider" class="Slide (strict)"("Visible"=w231) -> ()  [unwired: 2 in, 2 out]
            n127 = property on="Test Ring" class="Ring (strict)"("Visible"=w231) -> ()  [unwired: 2 in, 2 out]
            n128 = property on="Rev/Fwd" class="Clust (strict)"("Visible"=w231) -> ()  [unwired: 2 in, 2 out]
          }
          frame "Servo" {
            w247 = FALSE ("Visible")
            n129 = call <vilib>:"NT Read Number.vi"("Name"=w249) -> ("Numeric"=w248:dbl)  [unwired: 9 in, 1 out]
            n130 = property on="Test Slider" class="Slide (strict)"("Visible"=TRUE, "Scale.Maximum"=170.0 ("Scale.Range:Maximum")) -> ()  [unwired: 2 in, 2 out]
            n131 = local write "Test Slider"(w248) -> ()
            n132 = property on="Motor" class="Clust (strict)"("Visible"=w247) -> ()  [unwired: 2 in, 2 out]
            n133 = property on="Rev/Fwd" class="Clust (strict)"("Visible"=w247) -> ()  [unwired: 2 in, 2 out]
            n134 = property on="On/Off" class="Bool (strict)"("Visible"=w247) -> ()  [unwired: 2 in, 2 out]
            n135 = property on="Test Ring" class="Ring (strict)"("Visible"=w247) -> ()  [unwired: 2 in, 2 out]
          }
          frame "Relay", "Solenoid" {
            w250 = FALSE ("Visible")
            n136 = property on="Motor" class="Clust (strict)"("Visible"=w250) -> ()  [unwired: 2 in, 2 out]
            n137 = property on="Test Slider" class="Slide (strict)"("Visible"=w250) -> ()  [unwired: 2 in, 2 out]
            n138 = Search and Replace String(input string=w251, search string="/Value  **", replace string="/Direction") -> (result string=w257:string)  [unwired: 5 in, 3 out]
            n139 = property on="Test Ring" class="Ring (strict)"("Visible"=w250) -> ()  [unwired: 2 in, 2 out]
            n140 = call <vilib>:"NT Read String.vi"("Name"=w257) -> ("String"=w255:string)  [unwired: 9 in, 1 out]
            n141 = Equal?(x="Both directions", y=w255) -> (x = y?=w253:bool)
            n142 = Not(x=w253) -> (.not. x?=w254:bool)
            n143 = property on="Rev/Fwd" class="Clust (strict)"("Visible"=w253) -> ()  [unwired: 2 in, 2 out]
            n144 = property on="On/Off" class="Bool (strict)"("Visible"=w254, "Caption.Text"=w252) -> ()  [unwired: 2 in, 2 out]
          }
          frame "Compressor", "Digital Out" {
            w260 = FALSE ("Visible")
            # "Get direction and finish"
            n145 = property on="Motor" class="Clust (strict)"("Visible"=w260) -> ()  [unwired: 2 in, 2 out]
            n146 = property on="Test Slider" class="Slide (strict)"("Visible"=w260) -> ()  [unwired: 2 in, 2 out]
            n147 = property on="Test Ring" class="Ring (strict)"("Visible"=w260) -> ()  [unwired: 2 in, 2 out]
            n148 = property on="On/Off" class="Bool (strict)"("Visible"=TRUE, "Caption.Text"=w261) -> ()  [unwired: 2 in, 2 out]
            n149 = property on="Rev/Fwd" class="Clust (strict)"("Visible"=FALSE) -> ()  [unwired: 2 in, 2 out]
          }
          frame "Camera" {
            n150 = call <vilib>:"Get Last Path Segment.vi"("String in"=w268) -> ("String out"=w269:string)  [unwired: 10 in]
            n151 = property on="On/Off" class="Bool (strict)"("Visible"=FALSE) -> ()  [unwired: 2 in, 2 out]
            n152 = property on="Motor" class="Clust (strict)"("Visible"=FALSE) -> ()  [unwired: 2 in, 2 out]
            n153 = property on="Rev/Fwd" class="Clust (strict)"("Visible"=FALSE) -> ()  [unwired: 2 in, 2 out]
            n154 = case shown="\"White Balance  **\"" w269 {
              tunnel: w268 -> [w275 w284 w293 w302 w311 _ w317]
              tunnel: w267 -> [w273 w281 w290 w299 w308 _ _]
              frame "Size  **" {
                n155 = Index Array(array=w273) -> (element=w272:cluster{string[]})  [unwired: 1 in]
                n156 = call <vilib>:"NT Read String.vi"("Name"=w275) -> ("String"=w274:string)  [unwired: 9 in, 1 out]
                n157 = Unbundle(w272) -> (w270:string[])
                n158 = Match First String(2:w270, 3:w274) -> (0:w271:i32)  [unwired: 1 out]
                n159 = property on="Test Ring" class="Ring (strict)"("Value"=w271, "Strings []"=w270) -> ()  [unwired: 2 in, 2 out]
                n160 = property on="Test Ring" class="Ring (strict)"("Visible"=TRUE) -> ()  [unwired: 2 in, 2 out]
                n161 = property on="Test Slider" class="Slide (strict)"("Visible"=FALSE) -> ()  [unwired: 2 in, 2 out]
              }
              frame "White Balance  **" {
                n162 = Index Array(array=w281, index=1) -> (element=w282:cluster{string[]})
                n163 = call <vilib>:"NT Read String.vi"("Name"=w284) -> ("String"=w283:string)  [unwired: 9 in, 1 out]
                n164 = Unbundle(w282) -> (w279:string[])
                n165 = Match First String(2:w279, 3:w283) -> (0:w278:i32)  [unwired: 1 out]
                n166 = property on="Test Ring" class="Ring (strict)"("Value"=w278, "Strings []"=w279) -> ()  [unwired: 2 in, 2 out]
                n167 = property on="Test Ring" class="Ring (strict)"("Visible"=TRUE) -> ()  [unwired: 2 in, 2 out]
                n168 = property on="Test Slider" class="Slide (strict)"("Visible"=FALSE) -> ()  [unwired: 2 in, 2 out]
              }
              frame "Exposure  **" {
                n169 = Index Array(array=w290, index=2) -> (element=w291:cluster{string[]})
                n170 = call <vilib>:"NT Read String.vi"("Name"=w293) -> ("String"=w292:string)  [unwired: 9 in, 1 out]
                n171 = Unbundle(w291) -> (w287:string[])
                n172 = Match First String(2:w287, 3:w292) -> (0:w288:i32)  [unwired: 1 out]
                n173 = property on="Test Ring" class="Ring (strict)"("Value"=w288, "Strings []"=w287) -> ()  [unwired: 2 in, 2 out]
                n174 = property on="Test Ring" class="Ring (strict)"("Visible"=TRUE) -> ()  [unwired: 2 in, 2 out]
                n175 = property on="Test Slider" class="Slide (strict)"("Visible"=FALSE) -> ()  [unwired: 2 in, 2 out]
              }
              frame "Exposure Priority  **" {
                n176 = Index Array(array=w299, index=3) -> (element=w300:cluster{string[]})
                n177 = call <vilib>:"NT Read String.vi"("Name"=w302) -> ("String"=w301:string)  [unwired: 9 in, 1 out]
                n178 = Unbundle(w300) -> (w296:string[])
                n179 = Match First String(2:w296, 3:w301) -> (0:w297:i32)  [unwired: 1 out]
                n180 = property on="Test Ring" class="Ring (strict)"("Value"=w297, "Strings []"=w296) -> ()  [unwired: 2 in, 2 out]
                n181 = property on="Test Ring" class="Ring (strict)"("Visible"=TRUE) -> ()  [unwired: 2 in, 2 out]
                n182 = property on="Test Slider" class="Slide (strict)"("Visible"=FALSE) -> ()  [unwired: 2 in, 2 out]
              }
              frame "Color Enable  **" {
                n183 = Index Array(array=w308, index=4) -> (element=w309:cluster{string[]})
                n184 = call <vilib>:"NT Read String.vi"("Name"=w311) -> ("String"=w310:string)  [unwired: 9 in, 1 out]
                n185 = Unbundle(w309) -> (w305:string[])
                n186 = Match First String(2:w305, 3:w310) -> (0:w306:i32)  [unwired: 1 out]
                n187 = property on="Test Ring" class="Ring (strict)"("Value"=w306, "Strings []"=w305) -> ()  [unwired: 2 in, 2 out]
                n188 = property on="Test Ring" class="Ring (strict)"("Visible"=TRUE) -> ()  [unwired: 2 in, 2 out]
                n189 = property on="Test Slider" class="Slide (strict)"("Visible"=FALSE) -> ()  [unwired: 2 in, 2 out]
              }
              frame Default {
                n190 = property on="Test Ring" class="Ring (strict)"("Visible"=FALSE) -> ()  [unwired: 2 in, 2 out]
                n191 = property on="Test Slider" class="Slide (strict)"("Visible"=FALSE) -> ()  [unwired: 2 in, 2 out]
              }
              frame "Brightness  **", "Color Level  **", "Compression  **", "FPS  **", "Sharpness  **" {
                n192 = call <vilib>:"NT Read Number.vi"("Name"=w317) -> ("Numeric"=w316:dbl)  [unwired: 9 in, 1 out]
                n193 = local write "Test Slider"(w316) -> ()
                n194 = property on="Test Slider" class="Slide (strict)"("Visible"=TRUE, "Scale.Maximum"=100.0 ("Scale.Range:Maximum")) -> ()  [unwired: 2 in, 2 out]
                n195 = property on="Test Ring" class="Ring (strict)"("Visible"=FALSE) -> ()  [unwired: 2 in, 2 out]
              }
            }
          }
        }
        n196 = property on="Progress" class="Clust (strict)"("Visible"=FALSE) -> ()  [unwired: 2 in, 2 out]
      }
      event "Test Name": Mouse Enter {
        # "Populate the ring with the list of tests"
        n197 = event-data() -> ()  [unwired: 1 in, 1 out]
        n198 = call <vilib>:"NT Read String Array.vi"("Name"="/TestMode/TestList") -> ("String Array"=w326:string[])  [unwired: 9 in, 1 out]
        n199 = Build Array (concatenate)("Select the test to run...", w326) -> (w325:string[])
        n200 = property on="Test Name" class="Ring (strict)"("Strings []"=w325) -> ()  [unwired: 2 in, 2 out]
      }
      event "Test Name": Value Change {
        w329 = FALSE ("Visible")
        # "Tell the robot the test name to run"
        n201 = event-data() -> ("NewVal"=w333:u16)  [unwired: 1 in]
        n202 = property on="Test Name" class="Ring (strict)"() -> ("Strings []"=w334:string[])  [unwired: 2 in, 2 out]
        n203 = local write "Progress"(T7 {"Test Progress"=0, "Test Progress Text"=""} ("Progress")) -> ()
        n204 = Index Array(array=w334, index=w333) -> (element=w332:string)
        n205 = call <vilib>:"NT Write String.vi"("String"=w332, "Name"="/TestMode/TestName") -> ()  [unwired: 9 in, 1 out]
        n206 = property on="Progress" class="Clust (strict)"("Visible"=TRUE) -> ()  [unwired: 2 in, 2 out]
        n207 = property on="Motor" class="Clust (strict)"("Visible"=w329) -> ()  [unwired: 2 in, 2 out]
        n208 = property on="Test Slider" class="Slide (strict)"("Visible"=w329) -> ()  [unwired: 2 in, 2 out]
        n209 = property on="On/Off" class="Bool (strict)"("Visible"=w329) -> ()  [unwired: 2 in, 2 out]
        n210 = property on="Rev/Fwd" class="Clust (strict)"("Visible"=w329) -> ()  [unwired: 2 in, 2 out]
        n211 = property on="Test Ring" class="Ring (strict)"("Visible"=w329) -> ()  [unwired: 2 in, 2 out]
      }
      event "Select Auto": Mouse Enter {
        # "Populate the combo box with the list of autonomous options"
        n212 = event-data() -> ()  [unwired: 1 in, 1 out]
        n213 = call <vilib>:"NT Read String Array.vi"("Name"="Auto List") -> ("String Array"=w336:string[])  [unwired: 9 in, 1 out]
        n214 = property on="Select Auto" class="CmbBox"("Strings[]"=w336) -> ()  [unwired: 2 in, 2 out]
      }
      event "Select Auto": Value Change {
        # "User modified the Auto Selection. Write to NT variable so robot knows."
        n215 = event-data() -> ("NewVal"=w340:string)  [unwired: 1 in]
        n216 = call <vilib>:"NT Write String.vi"("String"=w340, "Name"="Auto Selector") -> ()  [unwired: 9 in, 1 out]
      }
      event "Command Selection": Value Change {
        # "Get the params and show in table"
        n217 = event-data() -> ("NewVal"=w347:i32)  [unwired: 1 in]
        n218 = property on="Command Selection" class="MCListbox (strict)"() -> ("ItemNames"=w345:string[][])  [unwired: 2 in, 2 out]
        n219 = call <vilib>:"WPI_DashboardUpdate Command Params.vi"("NewVal"=w347, "Commands"=w345, "Param Tbl"=w346) -> ()  [unwired: 8 in, 1 out]
      }
      event "Execute Command": Value Change {
        # "Started one, Unique ID holds\nresponse"
        n220 = event-data() -> ()  [unwired: 1 in, 1 out]
        n221 = property on="Command Selection" class="MCListbox (strict)"() -> ("ItemNames"=w359:string[][])  [unwired: 2 in, 2 out]
        n222 = Index Array(array=w359, index (row)="Command Selection", index (col)=0) -> (element=w357:string)
        n223 = call <vilib>:"Invoke Commands.vi"("Command Params"="Command Params", "Function Name"=w357) -> ("Params"=w353:u8, "Started"=w352:bool)  [unwired: 7 in, 1 out]
        n224 = Array Subset(array="Command Params", length (row)=w353) -> (w354:string[][])  [unwired: 3 in]
        n225 = Select(t="Executing" ("Cmd Status"), s=w352, f="" ("Cmd Status")) -> (s? t:f=→"Cmd Status":string)
      }
      event "Command Selection": Double Click {
        n226 = event-data() -> ("Row"=w369:i32)  [unwired: 1 in]
        n227 = property on="Command Selection" class="MCListbox (strict)"() -> ("ItemNames"=w372:string[][])  [unwired: 2 in, 2 out]
        n228 = local read "Command Params"() -> (w367:string[][])
        n229 = Index Array(array=w372, index (row)=w369, index (col)=0) -> (element=w370:string)
        n230 = call <vilib>:"Invoke Commands.vi"("Command Params"=w367, "Function Name"=w370) -> ("Params"=w366:u8, "Started"=w361:bool)  [unwired: 7 in, 1 out]
        n231 = Array Subset(array=w367, length (row)=w366) -> (w365:string[][])  [unwired: 3 in]
        n232 = Select(t="Executing" ("Cmd Status"), s=w361, f="" ("Cmd Status")) -> (s? t:f=w362:string)
        n233 = local write "Cmd Status"(w362) -> ()
      }
      event "CheckList": Double Click {
        # "Shift clears all"
        # "Update symbols on the listbox"
        n234 = event-data() -> ("PlatMods.Shift"=w375:bool, "Row"=w377:i32)  [unwired: 1 in]
        n235 = case shown="True" w375 {
          tunnel: w377 -> [w381 _]
          tunnel: 1 -> [w380 _]
          frame False {
            n236 = property on="CheckList" class="LstBox (strict)"() -> ("Item Symbols"=w379:i32[])  [unwired: 2 in, 2 out]
            n237 = Replace Array Subset(array=w379, new element=w380, index=w381) -> (w378:i32[])
            n238 = property on="CheckList" class="LstBox (strict)"("Item Symbols"=w378) -> ()  [unwired: 2 in, 2 out]
          }
          frame True {
            w382 = 0 ("Top Row")
            n239 = property on="CheckList" class="LstBox (strict)"() -> ("Number of Rows"=w384:u32)  [unwired: 2 in, 2 out]
            n240 = Initialize Array(0, w384) -> (w383:i32[])
            n241 = property on="CheckList" class="LstBox (strict)"("Top Row"=w382, "Value"=w382, "Item Symbols"=w383) -> ()  [unwired: 2 in, 2 out]
          }
        }
      }
      event "CheckList": Key Down {
        # "Update symbols on the listbox\nLeft and right keys check and uncheck"
        n242 = event-data() -> ("VKey"=w389:T22)  [unwired: 1 in]
        n243 = case shown="\"Left\", \"Right\"" w389 {
          selector: w389 -> [w394 _]
          tunnel: eventvkey."Left" ("VKey") -> [w392 _]
          frame "Left", "Right" {
            n244 = Equal?(x=w392, y=w394) -> (x = y?=w393:bool)
            n245 = Select(t=0, s=w393, f=1) -> (s? t:f=w395:i32)
            n246 = property on="CheckList" class="LstBox (strict)"() -> ("Item Symbols"=w398:i32[])  [unwired: 2 in, 2 out]
            n247 = Replace Array Subset(array=w398, new element=w395, index="CheckList") -> (w397:i32[])
            n248 = property on="CheckList" class="LstBox (strict)"("Item Symbols"=w397) -> ()  [unwired: 2 in, 2 out]
          }
          frame Default {
          }
        }
      }
      event "DB Camera Config": Value Change {
        # "Show or hide the cluster of controls, store in ini file"
        n249 = event-data() -> ("NewVal"=w403:bool)  [unwired: 1 in]
        n250 = case shown="False" w403 {
          tunnel: w402 -> [w412 _]
          tunnel: [w405 w423] -> w401
          tunnel: w400 -> [w404 w423]
          frame False {
            w419 = "Camera"
            w422 = FALSE ("Visible")
            n251 = local read "Camera Settings"() -> (w411:T2)
            n252 = Index Array(array=w412) -> (element=w415:cluster{string[]})  [unwired: 1 in]
            n253 = Unbundle(w411) -> ("Frame Rate"=w410:i32, "Compression"=w409:i32, "Size"=w413:u16)
            n254 = Unbundle(w415) -> (w414:string[])
            n255 = Index Array(array=w414, index=w413) -> (element=w408:string)
            n256 = call-poly <vilib>:"Write Key.vi"("section"=w419, "value"=w408, "key"="Size", "refnum"=w404) -> ("refnum out"=w421:T20)  [unwired: 2 in, 5 out]
            n257 = call-poly <vilib>:"Write Key.vi"("section"=w419, "value"=w410, "key"="FrameRate", "refnum"=w421) -> ("refnum out"=w420:T20)  [unwired: 1 in, 6 out]
            n258 = property on="Camera Settings" class="Clust (strict)"("Visible"=w422) -> ()  [unwired: 2 in, 2 out]
            n259 = local write "DB Camera Config"(w422) -> ()
            n260 = call-poly <vilib>:"Write Key.vi"("section"=w419, "value"=w409, "key"="Compression", "refnum"=w420) -> ("refnum out"=w406:T20)  [unwired: 1 in, 6 out]
            n261 = call <vilib>:"Close Config Data.vi"("refnum"=w406) -> ("file path"=w407:path)  [unwired: 2 in, 8 out]
            n262 = call <vilib>:"Open Config Data.vi"("configuration file path"=w407) -> ("refnum"=w405:T20)  [unwired: 8 in, 2 out]
          }
          frame True {
            n263 = property on="Camera Settings" class="Clust (strict)"("Visible"=TRUE) -> ()  [unwired: 2 in, 2 out]
          }
        }
      }
      event "Camera Settings": Value Change {
        # "Update summary string when any elements of DB camera change"
        n264 = event-data() -> ("NewVal"=w437:T2)  [unwired: 1 in]
        n265 = Index Array(array=w433) -> (element=w432:cluster{string[]})  [unwired: 1 in]
        n266 = Unbundle(w437) -> ("Frame Rate"=w428:i32, "Compression"=w427:i32, "Size"=w430:u16)
        n267 = Unbundle(w432) -> (w431:string[])
        n268 = Index Array(array=w431, index=w430) -> (element=w429:string)
        n269 = Format Into String(format string="%s   %dfps   %d%%", w429, w428, w427) -> (resulting string=w434:string)  [unwired: 2 in, 1 out]
        n270 = Build Array(w434) -> (w435:string[])
        n271 = property on="DB Camera Config" class="Bool (strict)"("Strings [4]"=w435) -> ()  [unwired: 2 in, 2 out]
      }
      event "Motor.Enable": Value Change {
        # "When the test mode otor enable helper is set, update that\ntree row item's value"
        n272 = event-data() -> ("NewVal"=w444:bool)  [unwired: 1 in]
        n273 = Unbundle("Motor") -> ("Value"=w443:dbl)  [unwired: 1 out]
        n274 = Select(t=w443, s=w444, f=0.0) -> (s? t:f=w441:dbl)
        n275 = call <vilib>:"NT Write Number.vi"("Numeric"=w441, "Name"=w440) -> ()  [unwired: 9 in, 1 out]
      }
      event "Test Slider": Value Change {
        # "When the test mode slider helper is set, update that\ntree row item's value"
        n276 = event-data() -> ("NewVal"=w448:dbl)  [unwired: 1 in]
        n277 = call <vilib>:"NT Write Number.vi"("Numeric"=w448, "Name"=w449) -> ()  [unwired: 9 in, 1 out]
      }
      event "On/Off": Value Change {
        # "When the test mode on/off helper value is set, update that\ntree row item's value"
        n278 = event-data() -> ("NewVal"=w454:bool)  [unwired: 1 in]
        n279 = Boolean To (0,1)(Boolean=w454) -> (0, 1=w453:i16)
        n280 = call <vilib>:"NT Write Number.vi"("Numeric"=w453, "Name"=w452) -> ()  [unwired: 9 in, 1 out]
      }
      event "Rev/Fwd": Value Change {
        # "When the test mode helper value for relays is set, update that\ntree row item's value"
        n281 = event-data() -> ("NewVal.Forward"=w463:bool, "NewVal.Reverse"=w462:bool)  [unwired: 1 in]
        n282 = Boolean To (0,1)(Boolean=w463) -> (0, 1=w459:i16)
        n283 = Boolean To (0,1)(Boolean=w462) -> (0, 1=w461:i16)
        n284 = Negate(x=w461) -> (-x=w460:i16)
        n285 = Add(x=w459, y=w460) -> (x+y=w458:i16)
        n286 = call <vilib>:"NT Write Number.vi"("Numeric"=w458, "Name"=w457) -> ()  [unwired: 9 in, 1 out]
      }
      event "Test Ring": Value Change {
        # "When a test mode helper value is selected from the ring,\nset the tree item's variable to the string value"
        n287 = event-data() -> ("NewVal"=w468:u16)  [unwired: 1 in]
        n288 = property on="Test Ring" class="Ring (strict)"() -> ("Strings []"=w469:string[])  [unwired: 2 in, 2 out]
        n289 = Index Array(array=w469, index=w468) -> (element=w467:string)
        n290 = call <vilib>:"NT Write String.vi"("String"=w467, "Name"=w466) -> ()  [unwired: 9 in, 1 out]
      }
      event "Rec Mode": Value Change {
        # "Update globals for recording mode and path to read log from.\nClear when logging and let NetworkTables set path for vision to\nuse."
        n291 = event-data() -> ("NewVal"=w481:enum32{"Stop", "Record", "Playback"})  [unwired: 1 in]
        n292 = global write "WPI_DashboardLogging Global.vi" "Logging Filename"(path "") -> ()
        n293 = global write "WPI_DashboardLogging Global.vi" "Recording"(w481) -> ()
        n294 = case shown="\"Playback\"" w481 {
          tunnel: w480 -> [_ w483 w492]
          tunnel: [_ _ w491] -> w477
          tunnel: [_ _ w490] -> _
          tunnel: w475 -> [_ _ w488]
          tunnel: cluster{i32, i32} {-250, 170} -> [_ _ w487]
          tunnel: [_ _ T23 {"Image Size"=TRUE, "Image Type"=TRUE, "Pixel Value"=TRUE, "ROI Information"=TRUE, "Zoom Factor"=FALSE} ("Image Information Shown:All Elements")] -> w473
          tunnel: [_ _ TRUE ("Zoom Factor")] -> w472
          tunnel: w471 -> [_ _ w484]
          frame Default {
          }
          frame "Stop", "Record" {
            # "Place Window too"
            n295 = invoke class="VI" method="FP.Close"(reference=w483) -> (reference out=w482:refnum<vi>)  [unwired: 2 in, 2 out]
            n296 = invoke class="VI" method="Abort VI"(reference=w482) -> ()  [unwired: 2 in, 3 out]
          }
          frame "Playback" {
            n297 = call "Open Playback Panel.vi"("Offset"=w487, "DB VI Ref"=w488, "Playback in"=w492) -> ("Playback out"=w489:refnum<vi>)  [unwired: 8 in]
            n298 = register-events(w489, w484) -> (reference out=w491:refnum<event-registration>, error out=w490:errorcluster)  [unwired: 2 in]
          }
        }
        n299 = property on="Camera Image" class="ImageControl"("Image Information Shown"=w473, "Image Information Visible"=w472) -> ()  [unwired: 2 in, 2 out]
        n300 = call <vilib>:"WPI_DashboardNT Log FieldName Cache.vi"("Operation"=enum16{"Lookup/Add", "Index", "Clear"}."Clear") -> ()  [unwired: 8 in, 3 out]
      }
      event Panel Close {
        w494 = enum32{"Stop", "Record", "Playback"}."Stop" ("Rec Mode")
        # "Playback window has been closed, abort"
        n301 = event-data() -> ()  [unwired: 1 in, 4 out]
        n302 = local write "Rec Mode"(w494) -> ()
        n303 = global write "WPI_DashboardLogging Global.vi" "Recording"(w494) -> ()
      }
      event Panel Close {
        # "Abort playback window and ourself"
        n304 = event-data() -> ()  [unwired: 1 in, 4 out]
        n305 = invoke class="VI" method="FP.Close"(reference=w500) -> (reference out=w499:refnum<vi>)  [unwired: 2 in, 2 out]
        n306 = invoke class="VI" method="Abort VI"(reference=w499) -> (error out=w498:errorcluster)  [unwired: 2 in, 2 out]
        n307 = invoke class="VI" method="Abort VI"(error in=w498) -> ()  [unwired: 2 in, 3 out]
      }
      event User Event {
        n308 = event-data() -> ("IDs"=w508:cluster{"RPC field ID":u16, "Unique ID":u16}, "String"=w507:string)  [unwired: 1 in]
        n309 = Bundle("IDs"=w508, "String"=w507) -> (w506:T9)  [unwired: 1 in]
        n310 = call <vilib>:"Retrieve RPC Response.vi"("RPC Response"=w506) -> ("Output"=w503:string[][])  [unwired: 10 in]
        n311 = Build Array (concatenate)(w501, w503) -> (w502:string[][])
        n312 = local write "Command Params"(w502) -> ()
        n313 = local write "Cmd Status"("" ("Cmd Status")) -> ()
      }
      event "Vision": Value Change {
        # "Enable/Disable Compression slider.\nHW USB is hard-coded into the camera"
        n314 = event-data() -> ("NewVal"=w515:u16)  [unwired: 1 in]
        n315 = Equal?(x=w515, y=u32 2 ("milliseconds to wait")) -> (x = y?=w513:bool)
        n316 = Select(t=T24."Disabled and Grayed Out" ("Disabled"), s=w513, f=T24."Enabled" ("Disabled")) -> (s? t:f=w510:T24)
        n317 = property on="Compression" class="Slide (strict)"("DisabledEnum"=w510) -> ()  [unwired: 2 in, 2 out]
      }
      event "Tree": Double Click {
        n318 = event-data() -> ("PlatMods"=w520:T27, "Tag"=w519:string)  [unwired: 1 in]
        n319 = Unbundle(w520) -> ("Shift"=w518:bool)  [unwired: 4 out]
        n320 = Not(x=w518) -> (.not. x?=w517:bool)
        n321 = call <vilib>:"NT Update Persistence.vi"("Persistence"=w517, "Name"=w519) -> ()  [unwired: 9 in, 1 out]
      }
    }
  }
  n322 = while {
    tunnel: w48 -> [w524]
    i -> [w527]
    stop <- FALSE stop-if-true
    n323 = Wait (ms)(milliseconds to wait=u32 100) -> ()  [unwired: 1 out]
    n324 = case shown="\"Playback\"" "Rec Mode" {
      tunnel: w527 -> [_ _ w542]
      tunnel: [u32 2829099 ("Base Color") u32 11141120 ("Target Color") w531] -> w523
      frame "Stop", Default {
        # "Reset the color, extra updates don't cost much"
      }
      frame "Record" {
      }
      frame "Playback" {
        # "Playback"
        n325 = Quotient & Remainder(x=w542, y=u32 50 ("milliseconds to wait")) -> (x-y*floor(x/y)=w538:u32)  [unwired: 1 out]
        n326 = Divide(x=w538, y=u32 50 ("milliseconds to wait")) -> (x/y=w535:dbl)
        n327 = Multiply(x=6.283185307179586, y=w535) -> (x*y=w540:dbl)
        n328 = Sine(x=w540) -> (sin(x)=w539:dbl)
        n329 = Absolute Value(x=w539) -> (abs(x)=w532:dbl)
        n330 = call "Interpolate RGB Color.vi"("Proportion"=w532, "Target Color"=u32 30976, "Base Color"=u32 2829099) -> ("Result Color"=w531:u32)  [unwired: 8 in]
      }
    }
    n331 = property class="Pane"(reference=w524, "PaneColor"=w523) -> ()  [unwired: 1 in, 2 out]
  }
  n332 = local write "Dashboard Tab"(T1."Drive" ("Dashboard Tab")) -> ()
  n333 = property on="On/Off" class="Bool (strict)"("Visible"=w16) -> ()  [unwired: 2 in, 2 out]
  n334 = property on="Motor" class="Clust (strict)"("Visible"=w16) -> ()  [unwired: 2 in, 2 out]
  n335 = property on="Progress" class="Clust (strict)"("Visible"=w16) -> ()  [unwired: 2 in, 2 out]
  n336 = property on="Test Ring" class="Ring (strict)"("Visible"=w16) -> ()  [unwired: 2 in, 2 out]
  n337 = property on="Rev/Fwd" class="Clust (strict)"("Visible"=w16) -> ()  [unwired: 2 in, 2 out]
  n338 = property on="Camera Settings" class="Clust (strict)"("Visible"=w16) -> ()  [unwired: 2 in, 2 out]
  n339 = local write "DB Camera Config"(w16) -> ()
  n340 = local write "Command Params"(string[][] [] ("Command Params")) -> ()
  n341 = while {
    tunnel: u16 1741 ("timeout ms (25000)") -> [w544]
    stop <- FALSE stop-if-true
    n342 = TCP Create Listener(10:w544) -> (0:w543:errorcluster, 3:w545:refnum<k5>)  [unwired: 4 in, 1 out]
    n343 = case shown="No Error" w543 {
      selector: w543 -> [w547 _]
      tunnel: w545 -> [w548 _]
      frame No Error {
        n344 = while {
          tunnel: w548 -> [w551]
          tunnel: w547 -> [w550]
          stop <- FALSE stop-if-true
          n345 = TCP Wait On Listener(8:w550, 11:w551) -> (0:w552:errorcluster, 4:w553:refnum<k5>)  [unwired: 2 in, 3 out]
          n346 = local write "TCP"(w553) -> ()
          n347 = case shown="No Error" w552 {
            frame No Error {
            }
            frame Error {
              n348 = Wait (ms)(milliseconds to wait=u32 1000) -> ()  [unwired: 1 out]
            }
          }
        }
      }
      frame Error {
        n349 = Wait (ms)(milliseconds to wait=u32 1000) -> ()  [unwired: 1 out]
      }
    }
  }
  n350 = global write "WPI_DashboardLogging Global.vi" "Recording"(w42) -> ()
  n351 = local write "Rec Mode"(w42) -> ()
  n352 = local write "Command Selection"(u16 0 ("milliseconds to wait")) -> ()
  n353 = call-poly <vilib>:"NT Read Value.vi"("Name"="Flip") -> ()  [unwired: 9 in, 2 out]
